vi "Actor Core.vi"(8 "error in":errorcluster, 11 "Preparation Line in":refnum<class "Preparation Line.lvclass">) -> (0 "error out":errorcluster, 3 "Actor out":refnum<class "Actor.lvclass">)   [LabVIEW 2015, in "cRIO-Carbondioxide.lvlib" / "CO2-Actor.lvlib" / "Preparation Line.lvclass"]
doc: "(<B>Filename</B>: Actor Framework.lvlib:Actor.lvclass:Actor Core.vi)\n\nReceives messages to the actor, reacts to them, and initiates any error handling that may shut the actor down.\n\nDescendant classes may override this VI to append parallel tasks for the actor to complete while it handles messages. Overrides use the Call Parent Method node."
uses:
  Preparation Line.lvclass
  <vilib>/ActorFramework/Actor/Actor.lvclass
  CO2 Actor/CO2 Actor.lvclass
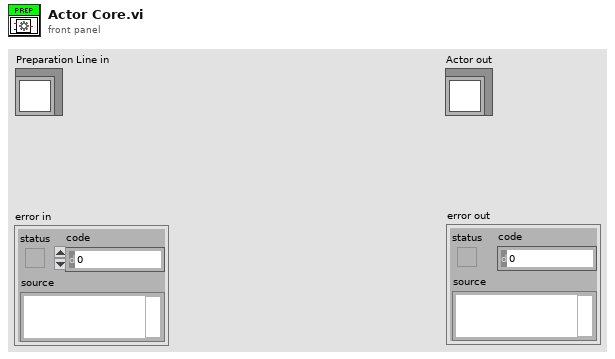
[diagram p1: front panel]
types:
  T1 = typedef "Sample Container.ctl" = cluster{"Sample In":refnum<k21>, "Sample Name":refnum<k21>, "Ti Cathode":refnum<k21>, "SampleQ":refnum<queue>}
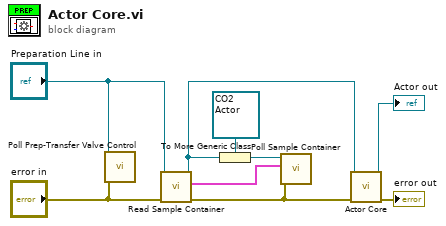
[diagram p0: block diagram]
diagram:
  n1 = call "Poll Prep-Transfer Valve Control.vi"("error in (no error)"="error in", "Preparation Line in"="Preparation Line in") -> ()  [unwired: 10 in]
  n2 = call "Read Sample Container.vi"("error in (no error)"="error in", "Preparation Line in"="Preparation Line in") -> ("error out"=w4:errorcluster, "Container"=w3:T1, "Preparation Line out"=w2:refnum<class "Preparation Line.lvclass">)  [unwired: 6 in, 1 out]
  n3 = To More Generic Class(target class=refnum<class "CO2 Actor.lvclass"> refnum ("CO2 Actor in"), reference=w2) -> (generic class reference=w1:refnum<class "CO2 Actor.lvclass">)
  n4 = call-dynamic "Poll Sample Container.vi"("error in (no error)"=w4, "Sample Container"=w3, "CO2 Actor in"=w1) -> ()  [unwired: 8 in, 1 out]
  n5 = call-parent "Actor Core.vi"("error in"=w4, "CO2 Actor in"=w2) -> ("error out"=→"error out":errorcluster, "Actor out"=→"Actor out":refnum<class "Actor.lvclass">)  [unwired: 8 in]
